vi "volgorde_kruispunten_deel2 (SubVI).vi"(10 "Numeric":dbl, 11 "OK Button":bool) -> (2 "Numeric 2":dbl)   [LabVIEW 2019]
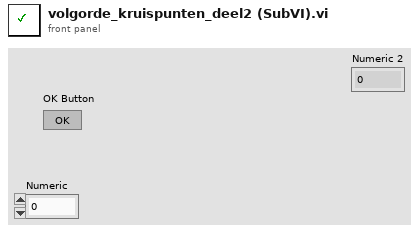
[diagram p1: front panel]
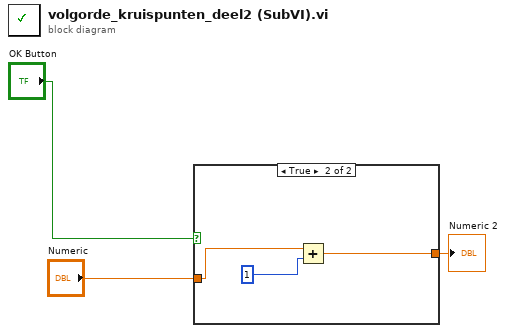
[diagram p0: block diagram]
diagram:
  n1 = case shown="True" "OK Button" {
    tunnel: "Numeric" -> [w4 w6]
    tunnel: [w4 w5] -> w1
    frame False {
    }
    frame True {
      n2 = Add(x=w6, y=1) -> (x+y=w5:dbl)
    }
  }
  "Numeric 2" <- w1
